vi "write image timmings.vi"(8 "error in (no error)":errorcluster, 11 "Save Image in":refnum<class "Save SPARC4 image.lvclass">) -> (0 "error out":errorcluster, 2 "timmings":T1, 3 "Save Image out":refnum<class "Save SPARC4 image.lvclass">)   [LabVIEW 2018, in "Save SPARC4 image.lvclass"]
uses:
  Save SPARC4 image.lvclass
  Save SPARC4 image.lvclass/Save SPARC4 image.ctl
  Channel/Channel.lvclass/Channel.ctl
  SPARC4_Channel/SPARC4_Channel.lvclass
  C:/Users/Denis/Desktop/S4ACS/S4ACS/Channel/Channel.lvclass
  Sim_CCD/Sim_CCD.lvclass
  Channel/Channel.lvclass
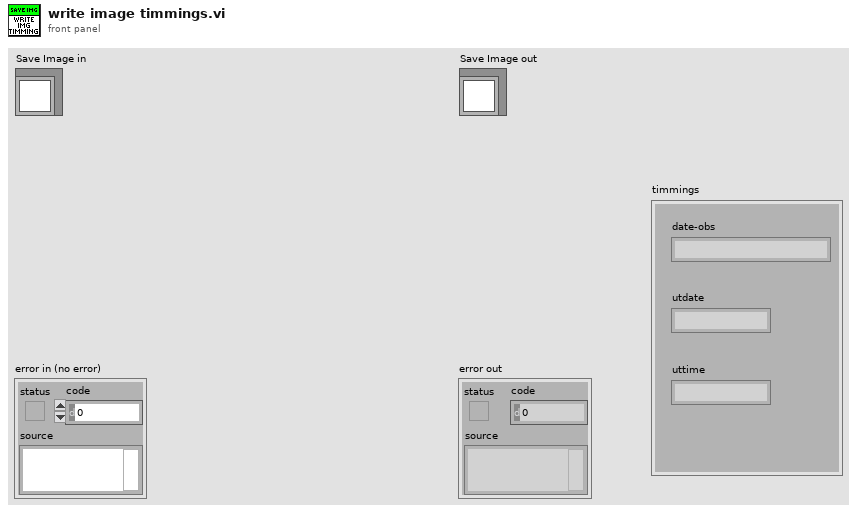
[diagram p1: front panel]
types:
  T1 = cluster{"date-obs":string, "utdate":string, "uttime":string}
  T2 = typedef "LVDateTimeRec.ctl" = cluster{"fractional second":dbl, "second":i32, "minute":i32, "hour":i32, "day of month":i32, "month":i32, "year":i32, "day of week":i32, "day of year":i32, "DST":i32}
  T3 = cluster{"Time Acq Started":u32, "Image delay":u64, "Last update - CCD config":timestamp, "SYSTEMTIME":T2, "Readout time":dbl, "Time acq finished":u32, "effective exptime":dbl}
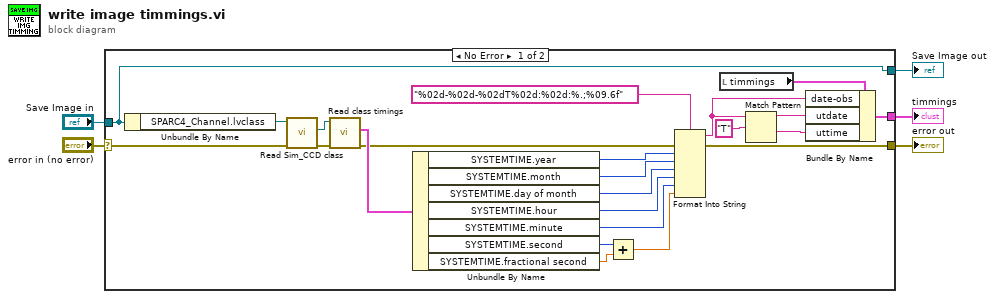
[diagram p0: block diagram]
diagram:
  n1 = case shown="No Error" "error in (no error)" {
    selector: "error in (no error)" -> [w20 w30]
    tunnel: [w6 w30] -> w4
    tunnel: [w21 w29] -> w2
    tunnel: "Save Image in" -> [w21 w29]
    tunnel: [w18 _] -> w1
    frame No Error {
      n2 = Unbundle By Name(w21) -> ("SPARC4_Channel.lvclass"=w22:refnum<class "SPARC4_Channel.lvclass">)
      n3 = call "Read Sim_CCD class.vi"("error in (no error)"=w20, "Channel in"=w22) -> ("error out"=w16:errorcluster, "Sim_CCD.lvclass"=w17:refnum<class "Sim_CCD.lvclass">)  [unwired: 7 in, 1 out]
      n4 = call "Read class timings.vi"("error in (no error)"=w16, "Simulated Camera in"=w17) -> ("error out"=w7:errorcluster, "class timings"=w15:T3)  [unwired: 7 in, 1 out]
      n5 = Unbundle By Name(w15) -> ("SYSTEMTIME.year"=w14:i32, "SYSTEMTIME.month"=w13:i32, "SYSTEMTIME.day of month"=w12:i32, "SYSTEMTIME.hour"=w11:i32, "SYSTEMTIME.minute"=w10:i32, "SYSTEMTIME.second"=w9:i32, "SYSTEMTIME.fractional second"=w8:dbl)
      n6 = Add(x=w9, y=w8) -> (x+y=w28:dbl)
      n7 = Format Into String(format string="%02d-%02d-%02dT%02d:%02d:%.;%09.6f", error in=w7, w14, w13, w12, w11, w10, w28) -> (resulting string=w27:string, error out=w6:errorcluster)  [unwired: 1 in]
      n8 = local read "timmings"() -> (w19:T1)
      n9 = Match Pattern(string=w27, regular expression="T") -> (before substring=w25:string, after substring=w23:string)  [unwired: 1 in, 2 out]
      n10 = Bundle By Name(cluster=w19, "date-obs"=w27, "utdate"=w25, "uttime"=w23) -> (w18:T1)
    }
    frame Error {
    }
  }
  "error out" <- w4
  "Save Image out" <- w2
  "timmings" <- w1
